vi "SCM1 He level.vi"() -> (11 "level warning":bool)   [LabVIEW 2025]
panel:
  out "Waveform Chart":waveform(dbl)(graph)
  in  "millisecond multiple":u32
  out "level":dbl
  out "error out":errorcluster
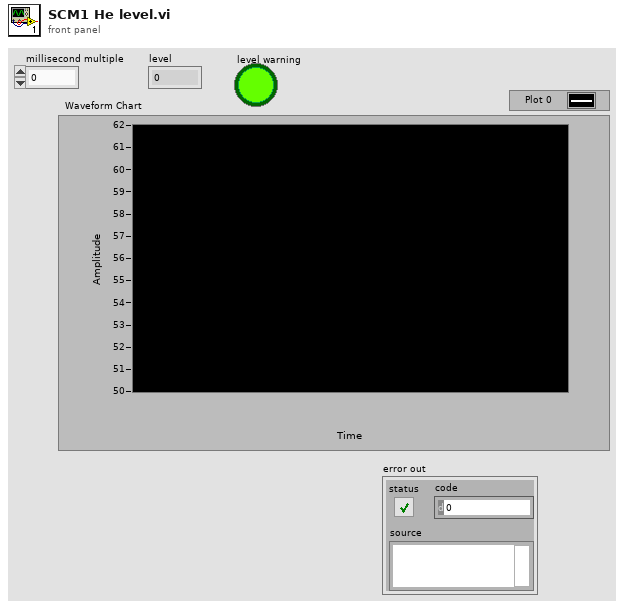
[diagram p1: front panel]
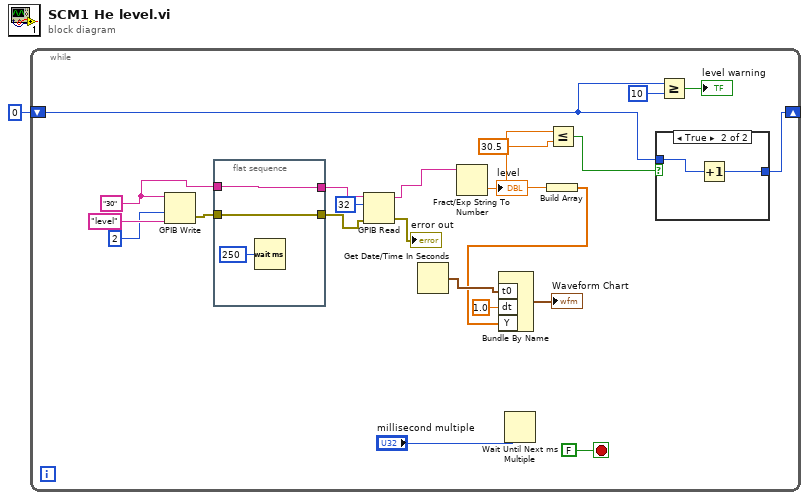
[diagram p0: block diagram]
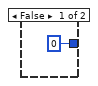
[diagram p2: hidden frame]
diagram:
  n1 = while {
    shift-right: [w5] -> _
    shift-left: u16 0 -> [w4]
    stop <- FALSE stop-if-true
    w17 = "30" ("address string")
    n2 = GPIB Write(0:w17, 1:"level" ("data"), 2:i16 2 ("mode (0)")) -> (6:w19:errorcluster)  [unwired: 2 in, 1 out]
    n3 = flat-sequence {
      tunnel: [w29] -> w20
      tunnel: w19 -> [w29]
      tunnel: w17 -> [w28]
      tunnel: [w28] -> w16
      frame #0 {
        n4 = Wait (ms)(milliseconds to wait=u32 250) -> ()  [unwired: 1 out]
      }
    }
    n5 = GPIB Read(0:w16, 1:32 ("byte count"), 3:w20) -> (5:w15:string, 7:→"error out":errorcluster)  [unwired: 2 in, 1 out]
    n6 = Get Date/Time In Seconds() -> (seconds since 1Jan1904=w11:timestamp)
    n7 = Fract/Exp String To Number(string=w15) -> (number=w8:dbl)  [unwired: 3 in, 1 out]
    "level" <- w8
    n8 = Wait Until Next ms Multiple(millisecond multiple="millisecond multiple") -> ()  [unwired: 1 out]
    n9 = Build Array(w8) -> (w9:dbl[])
    n10 = Bundle By Name("t0"=w11, "dt"=1.0, "Y"=w9) -> (→"Waveform Chart":waveform(dbl))  [unwired: 1 in]
    n11 = Less Or Equal?(x=w8, y=30.5) -> (x <= y?=w6:bool)
    n12 = case shown="True" w6 {
      tunnel: w4 -> [_ w26]
      tunnel: [u32 0 w25] -> w5
      frame False {
      }
      frame True {
        n13 = Increment(x=w26) -> (x+1=w25:u32)
      }
    }
    n14 = Greater Or Equal?(x=w4, y=u32 10) -> (x >= y?=→"level warning":bool)
  }
